vi "EnqueueMain.vi"(0 "object in":refnum<class "Application.lvclass">, 2 "Message":string, 3 "Message Data":variant, 5 "error in (no error)":errorcluster, 9 "Priority Message? (F)":bool) -> (14 "object out":refnum<class "Application.lvclass">, 19 "error out":errorcluster)   [LabVIEW 2019, in "Application.lvclass"]
uses:
  Application.lvclass
  Application.lvclass/Application.ctl
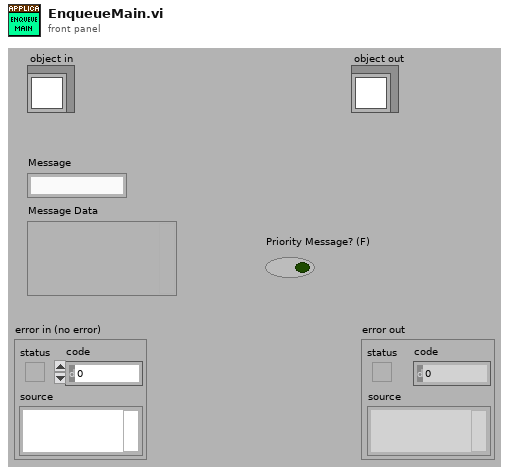
[diagram p1: front panel]
types:
  T1 = cluster{"Message":string, "Message Data":variant}
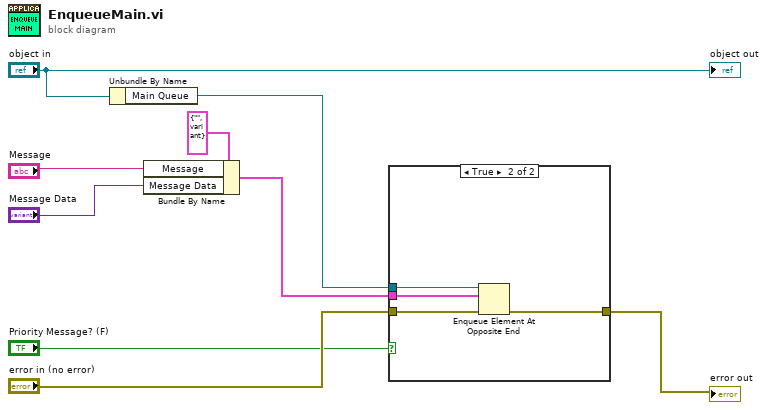
[diagram p0: block diagram]
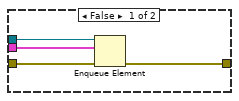
[diagram p2: hidden frame]
diagram:
  n1 = Unbundle By Name("object in") -> ("Main Queue"=w4:refnum<queue>)
  n2 = Bundle By Name(cluster=T1 {"Message"="", "Message Data"=variant} ("Message Cluster"), "Message"="Message", "Message Data"="Message Data") -> (w3:T1)
  n3 = case shown="True" "Priority Message? (F)" {
    tunnel: "error in (no error)" -> [w13 w17]
    tunnel: [w12 w16] -> w8
    tunnel: w4 -> [w11 w15]
    tunnel: w3 -> [w10 w14]
    frame False {
      n4 = Enqueue Element(queue=w11, element=w10, error in (no error)=w13) -> (error out=w12:errorcluster)  [unwired: 1 in, 2 out]
    }
    frame True {
      n5 = Enqueue Element At Opposite End(queue=w15, element=w14, error in (no error)=w17) -> (error out=w16:errorcluster)  [unwired: 1 in, 2 out]
    }
  }
  "error out" <- w8
  "object out" <- "object in"
